vi "DB Tools List Columns.vi"(4 "error in (no error)":errorcluster, 6 "table":string, 7 "connection reference":T3) -> (0 "error out":errorcluster, 1 "columns":string[](array[string]), 2 "column information":T2(array[cluster]), 3 "connection reference out":T3)   [LabVIEW 2017, in "NI_Database_API.lvlib"]
doc: "Lists the columns present in <B>table</B>. The column information includes the name, the data type, and the defined size of the column."
uses:
  <vilib>/addons/database/NI_Database_API.lvlib
  <vilib>/addons/database/Connection.llb/Conn ObjectReference.ctl
  <vilib>/addons/database/Auxilliary.llb/DB Tools DataTypes.ctl
  <vilib>/addons/database/Connection.llb/Conn Execute.vi
  <vilib>/addons/database/Recordset.llb/Rec Get Recordset Properties (R).vi
  <vilib>/addons/database/Recordset.llb/Rec Get Column Properties (R).vi
  <vilib>/addons/database/Recordset.llb/Rec Destroy - Connection.vi
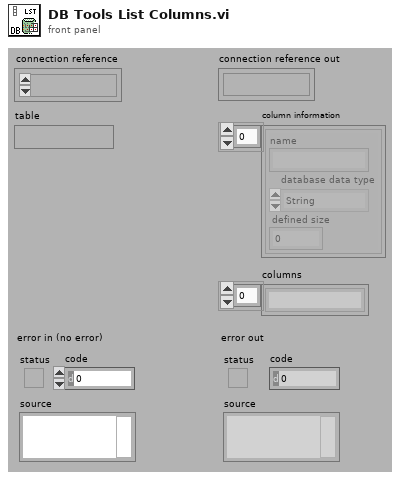
[diagram p1: front panel]
types:
  T1 = typedef "NI_Database_API.lvlib/DB Tools DataTypes.ctl" = enum16{"String", "Long (I32)", "Single (SGL)", "Double (DBL)", "Date/Time", "Binary"}
  T2 = cluster{"name":string, "database data type":T1, "defined size":i32}[]
  T3 = typedef "NI_Database_API.lvlib/Conn ObjectReference.ctl" = refnum<k1>
  T4 = cluster{"name":string, "database data type":enum16{"String", "Long (I32)", "Single (SGL)", "Double (DBL)", "Date/Time", "Binary"}, "defined size":i32}[]
  T5 = typedef "NI_Database_API.lvlib/Rec ObjectReference.ctl" = refnum<k1>
  T6 = typedef "NI_Database_API.lvlib/Rec Properties.ctl" = cluster{"column count":i32, "record index":i32, "record count":i32, "bof?":bool, "eof?":bool, "cursor type":T7, "cache size":i32, "state":enum16{"closed", "open"}}
  T7 = typedef "NI_Database_API.lvlib/DB Tools Cursor Type.ctl" = enum16{"forward-only", "keyset", "dynamic", "static"}
  T8 = typedef "NI_Database_API.lvlib/Rec Column Properties.ctl" = cluster{"name":string, "database data type":T1, "defined size":i32, "actual size":i32}
  T9 = cluster{"name":string, "database data type":T1, "defined size":i32}
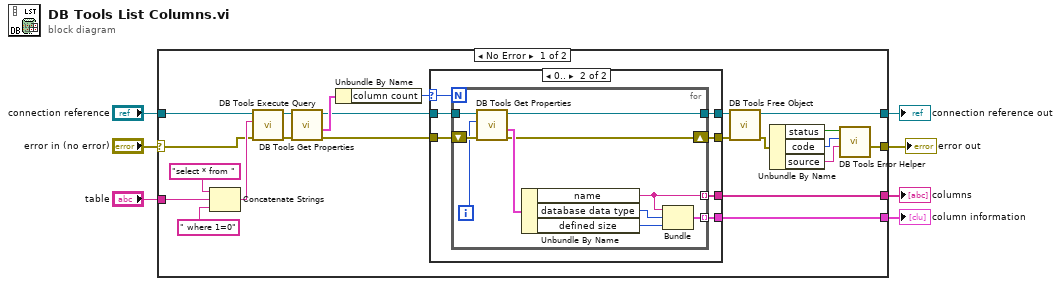
[diagram p0: block diagram]
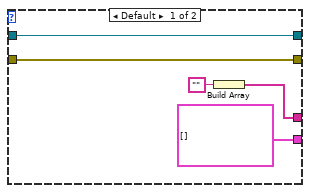
[diagram p2: hidden frame]
diagram:
  n1 = case shown="No Error" "error in (no error)" {
    selector: "error in (no error)" -> [w10 w53]
    tunnel: "connection reference" -> [w22 w52]
    tunnel: [w21 w52] -> w6
    tunnel: "table" -> [w19 _]
    tunnel: [w16 _] -> w4
    tunnel: [w15 _] -> w3
    tunnel: [w11 w53] -> w2
    frame No Error {
      n2 = Concatenate Strings("select * from " ("Substring"), w19, " where 1=0" ("Substring")) -> (w17:string)
      n3 = call-poly <vilib>:"DB Tools Execute Query.vi"("error in (no error)"=w10, "SQL query"=w17, "connection reference"=w22) -> ("error out"=w29:errorcluster, "recordset reference"=w28:T5)  [unwired: 5 in]
      n4 = call-poly <vilib>:"DB Tools Get Properties.vi"("error in (no error)"=w29, "recordset reference"=w28) -> ("error out"=w25:errorcluster, "recordset properties"=w27:T6, "recordset reference out"=w26:T5)  [unwired: 3 in]
      n5 = Unbundle By Name(w27) -> ("column count"=w8:i32)
      n6 = case shown="0.." w8 {
        selector: w8 -> [_ w35]
        tunnel: w26 -> [w34 w41]
        tunnel: w25 -> [w33 w40]
        tunnel: [w33 w39] -> w24
        tunnel: [w34 w38] -> w23
        tunnel: [T4 [] w37] -> w16
        tunnel: [w31 w36] -> w15
        frame Default {
          n7 = Build Array("") -> (w31:string[])
        }
        frame 0.. {
          n8 = for {
            N: w35 -> [_]
            tunnel: w41 -> [w50]
            shift-right: [w45] -> w39
            shift-left: w40 -> [w51]
            tunnel: [w46] -> w37 mode=indexing
            tunnel: [w44] -> w38
            tunnel: [w42] -> w36 mode=indexing
            i -> [w49]
            n9 = call-poly <vilib>:"DB Tools Get Properties.vi"("error in (no error)"=w51, "column index"=w49, "recordset reference"=w50) -> ("error out"=w45:errorcluster, "column properties"=w48:T8, "recordset reference out"=w44:T5)  [unwired: 2 in]
            n10 = Unbundle By Name(w48) -> ("name"=w42:string, "database data type"=w47:T1, "defined size"=w43:i32)
            n11 = Bundle("name"=w42, "database data type"=w47, "defined size"=w43) -> (w46:T9)  [unwired: 1 in]
          }
        }
      }
      n12 = call-poly <vilib>:"DB Tools Free Object.vi"("error in (no error)"=w24, "recordset reference"=w23) -> ("error out"=w12:errorcluster, "connection reference"=w21:T3)  [unwired: 8 in]
      n13 = Unbundle By Name(w12) -> ("status"=w13:bool, "code"=w9:i32, "source"=w14:string)
      n14 = call <vilib>:"DB Tools Error Helper.vi"("source"=w14, "code"=w9, "status"=w13) -> ("error out"=w11:errorcluster)  [unwired: 8 in]
    }
    frame Error {
    }
  }
  "connection reference out" <- w6
  "error out" <- w2
  "column information" <- w4
  "columns" <- w3
